vi "StatusUpdate.vi"(8 "error in (no error)":errorcluster, 9 "Status":string, 11 "Module":refnum<class "ModuleAdmin.lvclass">) -> (0 "error out":errorcluster, 3 "Module":refnum<class "ModuleAdmin.lvclass">)   [LabVIEW 2018, in "AcPwrPlugins.lvlib"]
doc: "This VI broadcasts a customized response for each request Main.vi received."
uses:
  AcPwrPlugins.lvlib
  <userlib>/NIST/ModuleAdminLib/ModuleAdmin/ModuleAdmin.lvclass
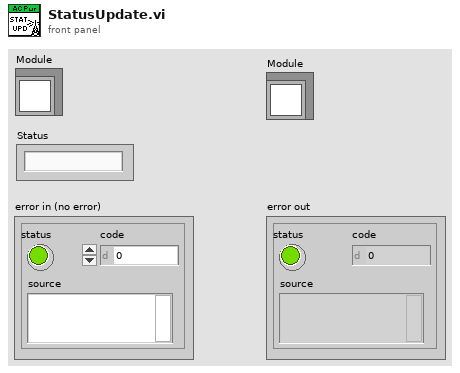
[diagram p1: front panel]
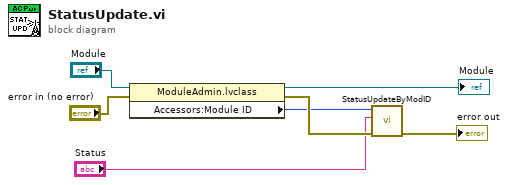
[diagram p0: block diagram]
diagram:
  n1 = property class="ModuleAdmin.lvclass"(reference="Module", error in="error in (no error)") -> (reference out=→"Module":refnum<class "ModuleAdmin.lvclass">, error out=w4:errorcluster, "Accessors:Module ID"=w2:i32)
  n2 = call "StatusUpdateByModID.vi"("error in (no error)"=w4, "Status"="Status", "Accessors:Module ID"=w2) -> ("error out"=→"error out":errorcluster)  [unwired: 8 in]
